vi "Aborts Dialog.vi"(8 "error in (no error)":errorcluster, 11 "Abort Parameters In":T2 {"Abort Criteria"."Comparison" items=["<", ">"]}) -> (0 "error out":errorcluster, 1 "Cancelled?":bool=TRUE, 2 "UI Refresh Needed?":bool, 3 "Abort Parameters Out":T2 {"Abort Criteria"."Comparison" items=["<", ">"]})   [LabVIEW 2024]
doc: "Dialog for selecting user specified settings."
uses:
  Abort Parameters.ctl
  23f40b91-b03b-4509-8bf9-68a1bf60e295.vi
  Display/Global 1.vi
  <vilib>/Utility/xml.llb/Write to XML File(string).vi
  <vilib>/Comparison/Equal/Equal Functor/Equal Functor.lvclass
panel:
  in  "Save as Preset":bool
  in  "Load Preset":bool
  in  "Abort Criteria":T1(array[cluster]) {"Comparison" items=["<", ">"]}
  in  "Sequence Duration":dbl
  in  "Sequence Delay":dbl
  in  "Cancel Button":bool
  in  "OK Button":bool
  # "Abort Parameters"
  # "Non visible portion of dialog (needed for connector pane)."
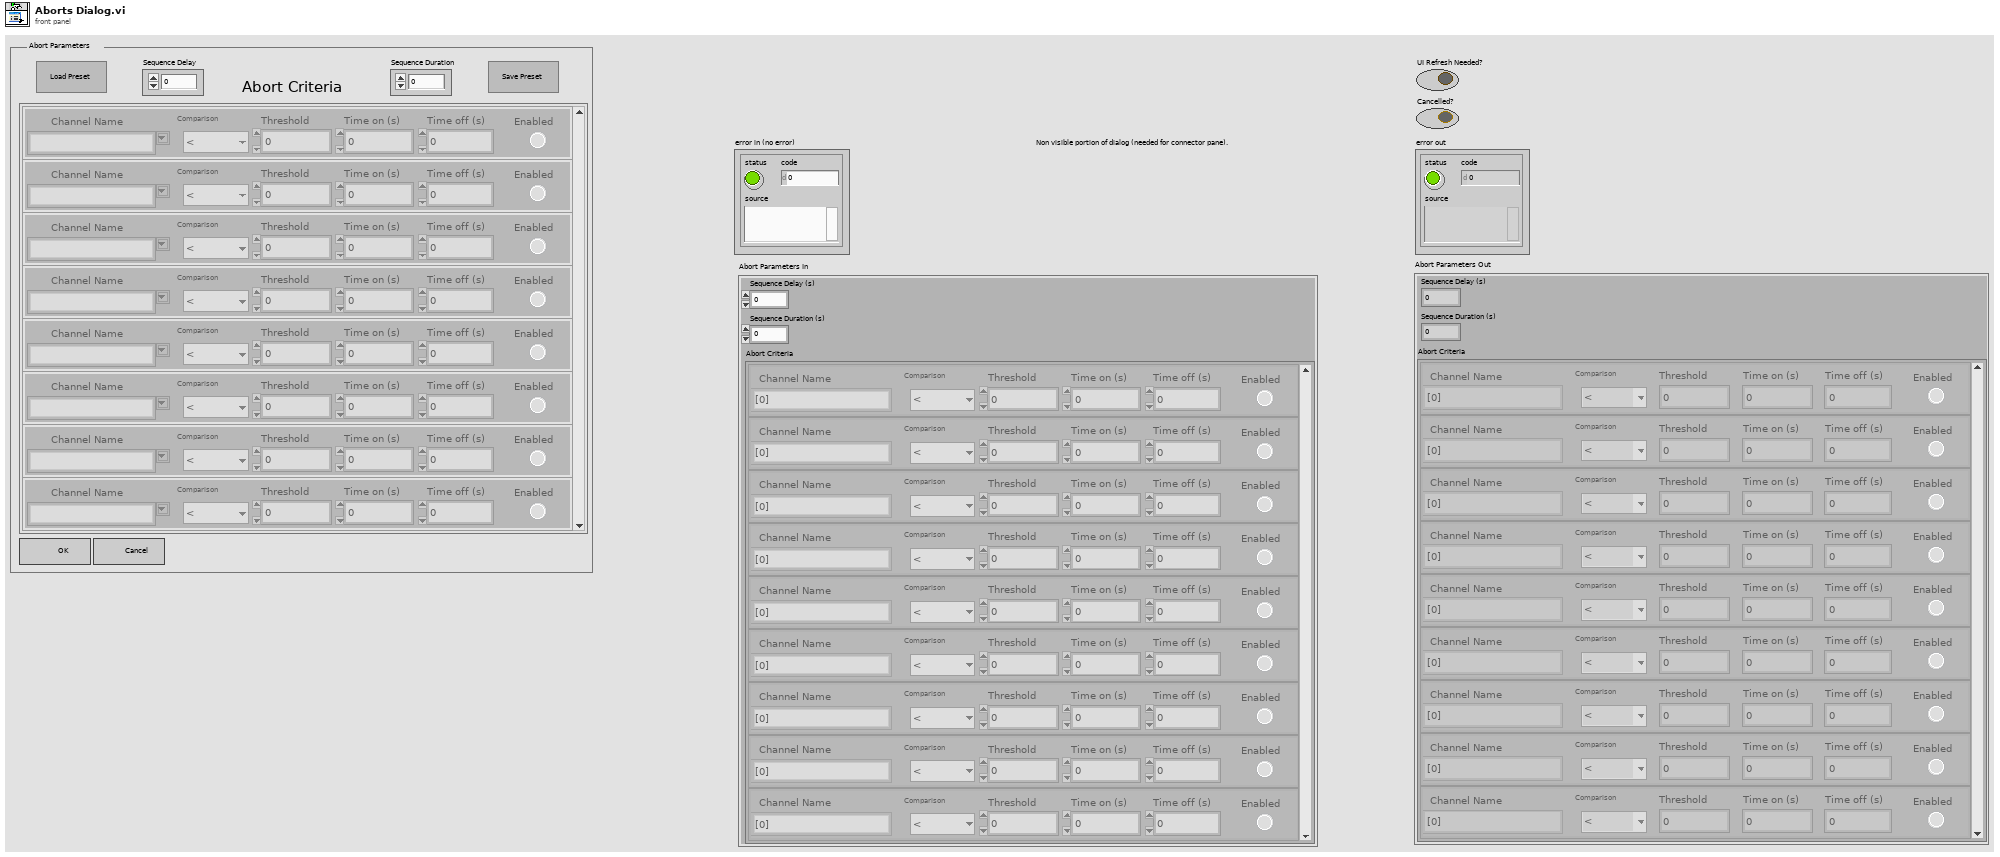
[diagram p1: front panel]
types:
  T1 = cluster{"Channel Name":string, "Comparison\n":u16, "Threshold":dbl, "Time on (s)":dbl, "Time off (s)":dbl, "Enabled":bool}[]
  T2 = typedef "Abort Parameters.ctl" = cluster{"Sequence Delay (s)":dbl, "Sequence Duration (s)":dbl, "Abort Criteria":cluster{"Channel Name\n":enum16{"[0]", "[1]", "[2]", "[3]", "[4]", "[5]", "[6]", "[7]", "[8]", "[9]", "[10]", "[11]", "[12]", "[13]", "[14]", "[15]", "[16]", "[17]", "[18]", "[19]", "[20]", "[21]", "[22]", "[23]", "[24]", "[25]", "[26]", "[27]", "[28]", "[29]", "[30]", "[31]", "[32]", "[33]", "[34]", "[35]", "[36]", "[37]", "[38]", "[39]", "[40]", "[41]", "[42]", "[43]", "[44]", "[45]", "[46]", "[47]", "[48]", "[49]"}, "Comparison\n":u16, "Threshold":dbl, "Time on (s)":dbl, "Time off (s)":dbl, "Enabled":bool}[]}
  T3 = typedef "Calibration Configuration.ctl" = cluster{"ai Calibration Slope":dbl[], "ai Calibration Offset":dbl[], "ai Sensor Names ":string[], "tc Sensor Names":string[], "di Sensor Names":string[], "do Sensor Names":string[], "bc Sensor Names":string[], "ai Sensor Units":string[], "tc Sensor Units":string[], "bc Sensor Units":string[]}
  T4 = cluster{"Channel Name\n":enum16{"[0]", "[1]", "[2]", "[3]", "[4]", "[5]", "[6]", "[7]", "[8]", "[9]", "[10]", "[11]", "[12]", "[13]", "[14]", "[15]", "[16]", "[17]", "[18]", "[19]", "[20]", "[21]", "[22]", "[23]", "[24]", "[25]", "[26]", "[27]", "[28]", "[29]", "[30]", "[31]", "[32]", "[33]", "[34]", "[35]", "[36]", "[37]", "[38]", "[39]", "[40]", "[41]", "[42]", "[43]", "[44]", "[45]", "[46]", "[47]", "[48]", "[49]"}, "Comparison\n":u16, "Threshold":dbl, "Time on (s)":dbl, "Time off (s)":dbl, "Enabled":bool}[]
  T5 = enum16{"[0]", "[1]", "[2]", "[3]", "[4]", "[5]", "[6]", "[7]", "[8]", "[9]", "[10]", "[11]", "[12]", "[13]", "[14]", "[15]", "[16]", "[17]", "[18]", "[19]", "[20]", "[21]", "[22]", "[23]", "[24]", "[25]", "[26]", "[27]", "[28]", "[29]", "[30]", "[31]", "[32]", "[33]", "[34]", "[35]", "[36]", "[37]", "[38]", "[39]", "[40]", "[41]", "[42]", "[43]", "[44]", "[45]", "[46]", "[47]", "[48]", "[49]"}
  T6 = cluster{"di Sensor":string, "Comparison\n":u16, "Threshold":dbl, "Time on (s)":dbl, "Time off (s)":dbl, "Enabled":bool}
  T7 = cluster{"index of element":i32, "Comparison\n":u16, "Threshold":dbl, "Time on (s)":dbl, "Time off (s)":dbl, "Enabled":bool}
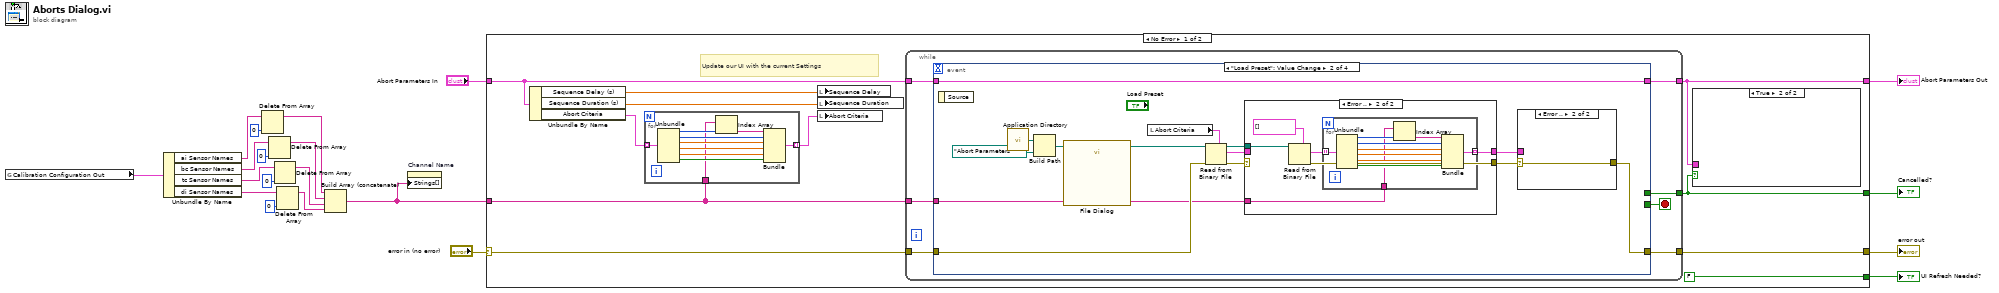
[diagram p0: block diagram]
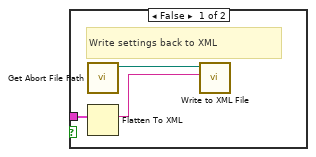
[diagram p2: hidden frame]
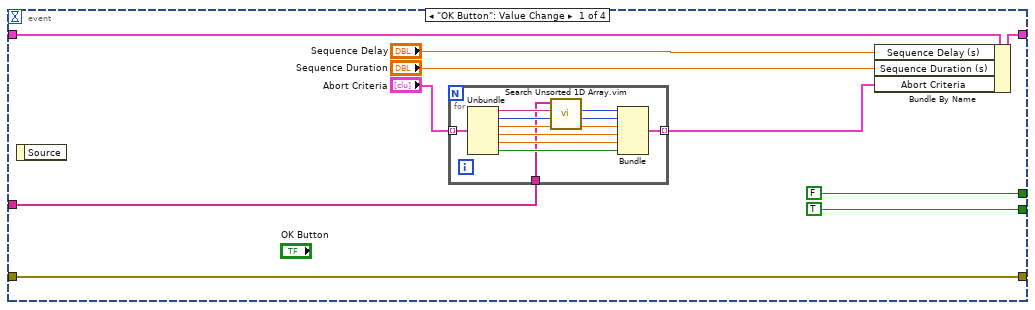
[diagram p3: hidden frame]
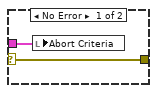
[diagram p4: hidden frame]
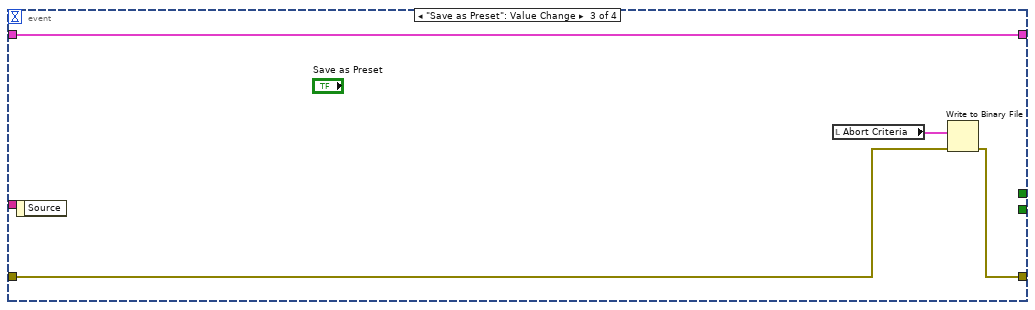
[diagram p6: hidden frame]
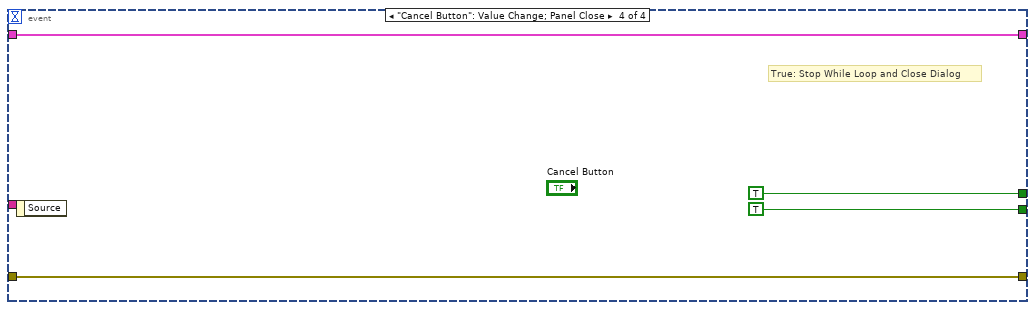
[diagram p7: hidden frame]
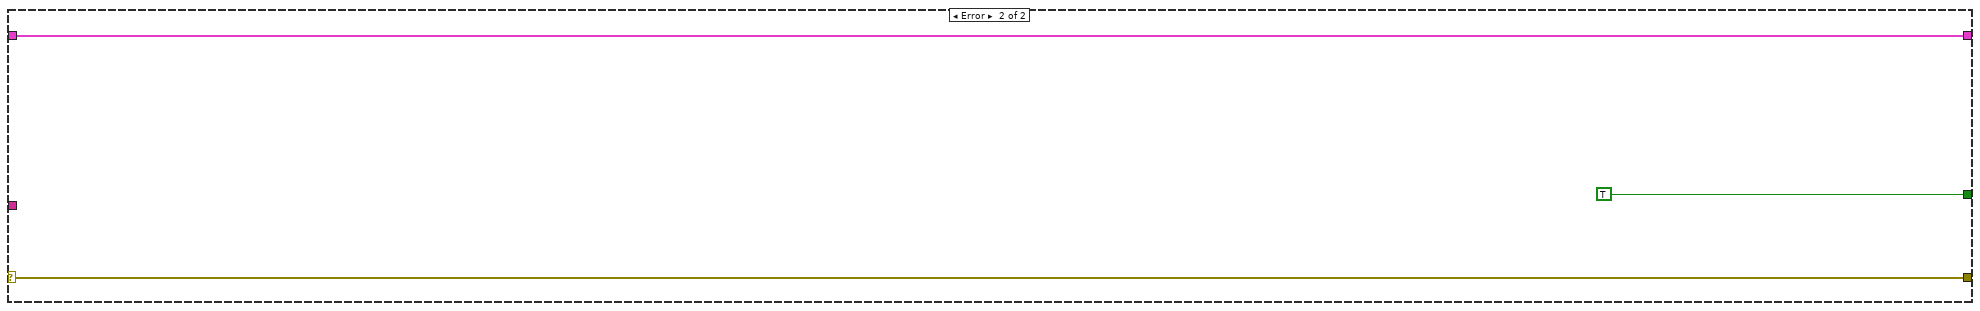
[diagram p8: hidden frame]
diagram:
  n1 = global read "Global 1.vi" "Calibration Configuration Out"() -> (w2:T3)
  n2 = Unbundle By Name(w2) -> ("ai Sensor Names"=w4:string[], "bc Sensor Names"=w12:string[], "tc Sensor Names"=w10:string[], "di Sensor Names"=w8:string[])
  n3 = Delete From Array(array=w4, index=0) -> (array with subset deleted=w3:string[])  [unwired: 1 in, 1 out]
  n4 = Delete From Array(array=w12, index=0) -> (array with subset deleted=w7:string[])  [unwired: 1 in, 1 out]
  n5 = Delete From Array(array=w10, index=0) -> (array with subset deleted=w6:string[])  [unwired: 1 in, 1 out]
  n6 = Delete From Array(array=w8, index=0) -> (array with subset deleted=w5:string[])  [unwired: 1 in, 1 out]
  n7 = Build Array (concatenate)(w3, w7, w6, w5) -> (w1:string[])
  n8 = property on="Channel Name" class="CmbBox"("Strings[]"=w1) -> ()  [unwired: 2 in, 2 out]
  n9 = case shown="No Error" "error in (no error)" {
    selector: "error in (no error)" -> [w25 w116]
    tunnel: [w24 w116] -> w20
    tunnel: "Abort Parameters In" -> [w30 w115]
    tunnel: [w27 w115] -> w15
    tunnel: [FALSE ("UI Refresh Needed?") _] -> w19
    tunnel: [w26 TRUE ("UI Refresh Needed?")] -> w18
    tunnel: w1 -> [w21 _]
    frame No Error {
      # "Update our UI with the current Settings"
      n10 = Unbundle By Name(w30) -> ("Sequence Delay (s)"=w29:dbl, "Sequence Duration (s)"=w28:dbl, "Abort Criteria"=w23:T4)
      n11 = for {
        tunnel: w23 -> [w41] mode=indexing
        tunnel: [w40] -> w22 mode=indexing
        tunnel: w21 -> [w32]
        n12 = Unbundle(w41) -> ("Channel Name"=w33:T5, "Comparison"=w39:u16, "Threshold"=w38:dbl, "Time on (s)"=w37:dbl, "Time off (s)"=w36:dbl, "Enabled"=w35:bool)
        n13 = Index Array(array=w32, index=w33) -> (element=w34:string)
        n14 = Bundle("di Sensor"=w34, "Comparison"=w39, "Threshold"=w38, "Time on (s)"=w37, "Time off (s)"=w36, "Enabled"=w35) -> (w40:T6)  [unwired: 1 in]
      }
      n15 = local write "Sequence Delay"(w29) -> ()
      n16 = local write "Sequence Duration"(w28) -> ()
      n17 = local write "Abort Criteria"(w22) -> ()
      n18 = while {
        tunnel: [w51] -> w26
        tunnel: [w50] -> w27
        tunnel: w30 -> [w49]
        tunnel: w25 -> [w47]
        tunnel: [w46] -> w24
        tunnel: w21 -> [w45]
        stop <- w48 stop-if-true
        n19 = event shown="[1] \"Load Preset\": Value Change" {
          selector: _ -> [_ _ _ _]
          dyn-events: _ -> [_ _ _ _]
          timeout: _ -> [_ _ _ _]
          tunnel: [w58 w83 w109 w113] -> w50
          tunnel: w49 -> [w59 w83 w109 w113]
          tunnel: [FALSE ("UI Refresh Needed?") _ _ TRUE ("UI Refresh Needed?")] -> w51
          tunnel: [TRUE _ _ TRUE] -> w48
          tunnel: w47 -> [w55 w84 w108 w110]
          tunnel: [w55 w79 w107 w110] -> w46
          tunnel: w45 -> [w52 w76 _ _]
          event "OK Button": Value Change {
            n20 = event-data() -> ()  [unwired: 1 in, 1 out]
            n21 = for {
              tunnel: "Abort Criteria" -> [w71] mode=indexing
              tunnel: [w70] -> w53 mode=indexing
              tunnel: w52 -> [w62]
              n22 = Unbundle(w71) -> ("Channel Name"=w63:string, "Comparison"=w69:u16, "Threshold"=w68:dbl, "Time on (s)"=w67:dbl, "Time off (s)"=w66:dbl, "Enabled"=w65:bool)
              n23 = call "Search Unsorted 1D Array.vim"("element"=w63, "unsorted 1D array"=w62) -> ("index of element"=w64:i32)  [unwired: 9 in]
              n24 = Bundle("index of element"=w64, "Comparison"=w69, "Threshold"=w68, "Time on (s)"=w67, "Time off (s)"=w66, "Enabled"=w65) -> (w70:T7)  [unwired: 1 in]
            }
            n25 = Bundle By Name(cluster=w59, "Sequence Delay (s)"="Sequence Delay", "Sequence Duration (s)"="Sequence Duration", "Abort Criteria"=w53) -> (w58:T2)
          }
          event "Load Preset": Value Change {
            n26 = event-data() -> ()  [unwired: 1 in, 1 out]
            n27 = call <vilib>:"Application Directory.vi"() -> ("Application Directory"=w74:path)
            n28 = Build Path(base path=w74, name or relative path=path "Abort Parameters") -> (appended path=w72:path)
            n29 = call "File Dialog"("start path"=w72) -> ("selected path"=w75:path)  [unwired: 11 in, 3 out]
            n30 = local read "Abort Criteria"() -> (w82:T1)
            n31 = Read from Binary File(5:w82, 8:w84, 11:w75) -> (0:w81:errorcluster, 2:w78:T1)  [unwired: 3 in, 2 out]
            n32 = case shown="Error .." w81 {
              selector: w81 -> [w89 _]
              tunnel: [w89 w95] -> w80
              tunnel: w78 -> [w88 _]
              tunnel: [w88 w93] -> w77
              tunnel: w76 -> [_ w92]
              tunnel: w75 -> [_ w90]
              frame No Error {
              }
              frame Error {
                n33 = Read from Binary File(5:T4 [] ("Abort Criteria"), 11:w90) -> (0:w95:errorcluster, 2:w94:T4)  [unwired: 4 in, 2 out]
                n34 = for {
                  tunnel: w94 -> [w105] mode=indexing
                  tunnel: [w104] -> w93 mode=indexing
                  tunnel: w92 -> [w96]
                  n35 = Unbundle(w105) -> ("Channel Name"=w97:T5, "Comparison"=w103:u16, "Threshold"=w102:dbl, "Time on (s)"=w101:dbl, "Time off (s)"=w100:dbl, "Enabled"=w99:bool)
                  n36 = Index Array(array=w96, index=w97) -> (element=w98:string)
                  n37 = Bundle("di Sensor"=w98, "Comparison"=w103, "Threshold"=w102, "Time on (s)"=w101, "Time off (s)"=w100, "Enabled"=w99) -> (w104:T6)  [unwired: 1 in]
                }
              }
            }
            n38 = case shown="Error .." w80 {
              selector: w80 -> [w85 w87]
              tunnel: w77 -> [w86 _]
              tunnel: [w85 w87] -> w79
              frame No Error {
                n39 = local write "Abort Criteria"(w86) -> ()
              }
              frame Error {
              }
            }
          }
          event "Save as Preset": Value Change {
            n40 = event-data() -> ()  [unwired: 1 in, 1 out]
            n41 = local read "Abort Criteria"() -> (w106:T1)
            n42 = Write to Binary File(data=w106, error in=w108) -> (error out=w107:errorcluster)  [unwired: 4 in, 2 out]
          }
          event "Cancel Button": Value Change; Panel Close {
            # "True: Stop While Loop and Close Dialog"
            n43 = event-data() -> ()  [unwired: 1 in, 1 out]
          }
        }
      }
      n44 = case shown="True" w26 {
        tunnel: w27 -> [w44 _]
        frame False {
          # "Write settings back to XML"
          n45 = call "Get Abort File Path.vi"() -> ("XML File Path"=w42:path)  [unwired: 10 in, 1 out]
          n46 = Flatten To XML(6:w44) -> (2:w43:string)
          n47 = call-poly <vilib>:"Write to XML File.vi"("XML Input"=w43, "XML File Path"=w42) -> ()  [unwired: 7 in, 3 out]
        }
        frame True {
        }
      }
    }
    frame Error {
    }
  }
  "UI Refresh Needed?" <- w19
  "error out" <- w20
  "Cancelled?" <- w18
  "Abort Parameters Out" <- w15
